vi "Add Correction.vi"(8 "error in (no error)":errorcluster, 9 "Type of Hexaboard":T1, 10 "XYZTheta":dbl[](array[numeric]), 11 "Carrier Tray in":refnum<class "Assembly Tray.lvclass">) -> (0 "error out":errorcluster, 2 "XYZTheta Out":dbl[](array[numeric]), 3 "Carrier Tray out":refnum<class "Assembly Tray.lvclass">)   [LabVIEW 2021, in "Assembly Tray.lvclass"]
uses:
  Assembly Tray.lvclass
  C:/Users/hep/Documents/UCSB-CMU-GantryCode/UCSB-Gantry-HEP-main (3)/UCSB-Gantry-HEP-main/Classes/Workspace/Fixture.lvclass
  Routine/TypeOfHexaboard.ctl
  Fixture.lvclass/Fixture.ctl
  Read Fixture ID.vi
  Read Position.vi
  Routine/Routine.lvclass
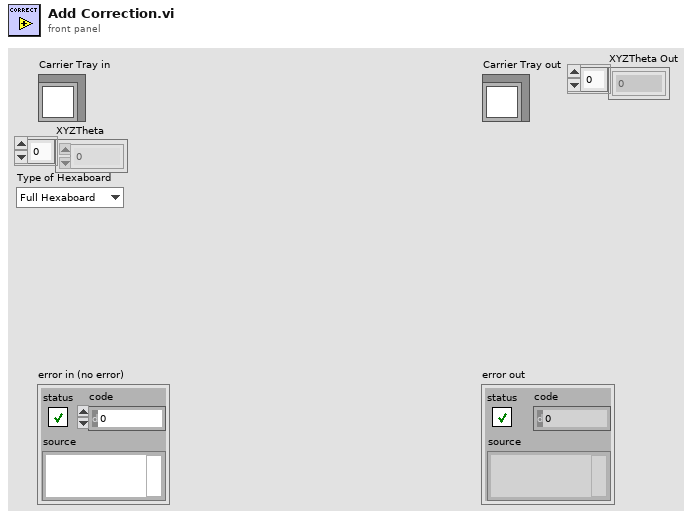
[diagram p1: front panel]
types:
  T1 = typedef "Routine.lvclass/TypeOfHexaboard.ctl" = enum16{"Full Hexaboard", "Right Partial PCB", "Right Partial Sensor", "Al Dummy Right Partial Sensor"}
  T2 = typedef "File Paths.ctl" = cluster{"Glue Pattern Folder":path, "Carrier Tray Folder":path, "Pick Up Tool Fixture Folder":path, "Components Folder":path, "Bellows Tool Offset.txt":path, "Pick Up Tool Offset.txt":path, "Dispense Tip Offset.txt":path, "Log Files":path, "Gantry Assembly Map.txt":path, "Syringe and offset map.txt":path}
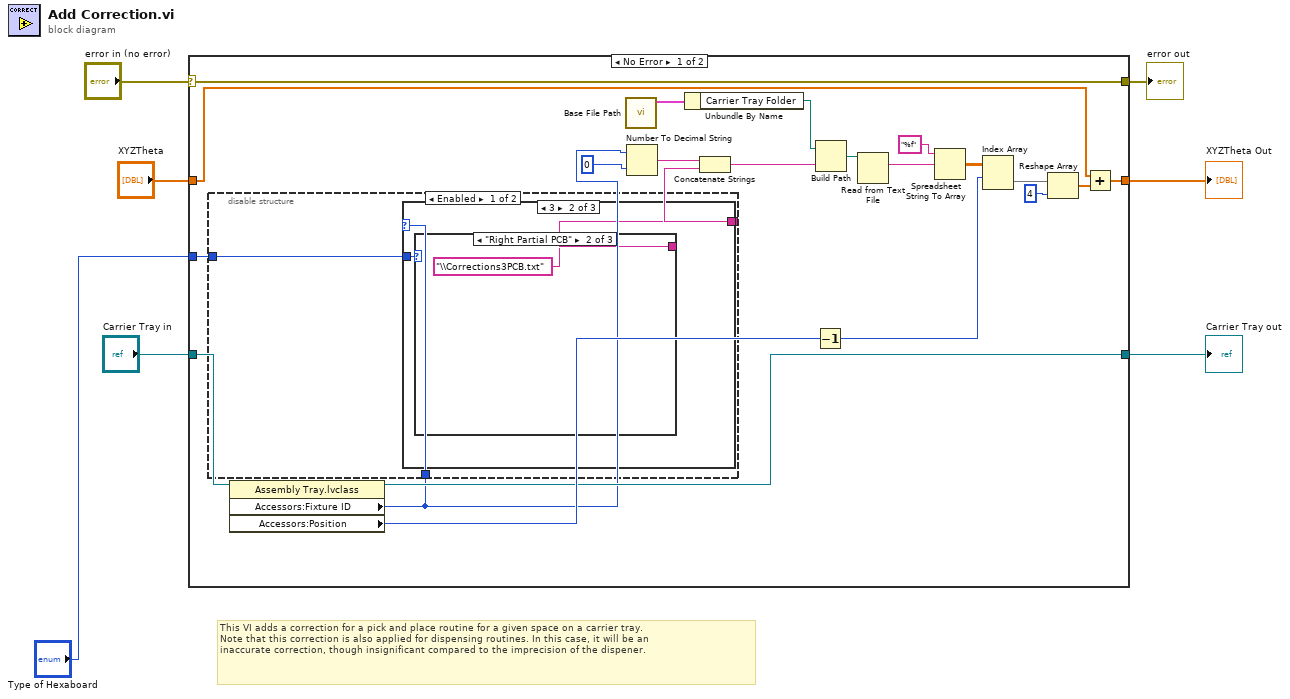
[diagram p0: block diagram]
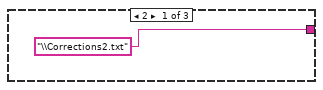
[diagram p2: hidden frame]
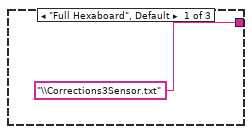
[diagram p3: hidden frame]
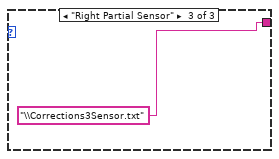
[diagram p4: hidden frame]
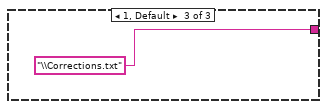
[diagram p5: hidden frame]
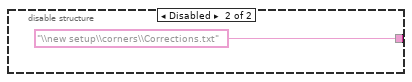
[diagram p6: hidden frame]
diagram:
  # "This VI adds a correction for a pick and place routine for a given space on a carrier tray.\nNote that this correction is also applied for dispensing routines. In this case, it will be an\ninaccurate correction, though insignificant compared to the imprecision of the dispener."
  n1 = case shown="No Error" "error in (no error)" {
    selector: "error in (no error)" -> [w29 w43]
    tunnel: [w29 w43] -> w6
    tunnel: [w10 w42] -> w4
    tunnel: "Carrier Tray in" -> [w12 w42]
    tunnel: "XYZTheta" -> [w15 w41]
    tunnel: [w13 w41] -> w2
    tunnel: "Type of Hexaboard" -> [w8 _]
    frame No Error {
      n2 = property class="Assembly Tray.lvclass"(reference=w12) -> (reference out=w10:refnum<class "Assembly Tray.lvclass">, "Accessors:Fixture ID"=w9:i32, "Accessors:Position"=w11:i32)  [unwired: 1 in, 1 out]
      n3 = disable-structure shown="Enabled" {
        disable-tunnel: [w32 "\\new setup\\corners\\Corrections.txt" ("name or relative path")] -> w24
        disable-tunnel: w9 -> [w31 _]
        disable-tunnel: w8 -> [w30 _]
        frame Enabled {
          n4 = case shown="3" w31 {
            tunnel: ["\\Corrections2.txt" ("name or relative path") w35 "\\Corrections.txt" ("name or relative path")] -> w32
            tunnel: w30 -> [_ w34 _]
            frame 2 {
            }
            frame 3 {
              n5 = case shown="\"Right Partial PCB\"" w34 {
                tunnel: ["\\Corrections3Sensor.txt" ("name or relative path") "\\Corrections3PCB.txt" ("name or relative path") "\\Corrections3Sensor.txt" ("name or relative path")] -> w35
                frame "Full Hexaboard", Default {
                }
                frame "Right Partial PCB" {
                }
                frame "Right Partial Sensor" {
                }
              }
            }
            frame 1, Default {
            }
          }
        }
        frame Disabled {
        }
      }
      n6 = call "Base File Path.vi"() -> ("Paths Out"=w28:T2)  [unwired: 11 in]
      n7 = Number To Decimal String(number=w9, width (-)=i16 0) -> (decimal integer string=w25:string)
      n8 = Unbundle By Name(w28) -> ("Carrier Tray Folder"=w27:path)
      n9 = Concatenate Strings(w25, w24) -> (w23:string)
      n10 = Decrement(x=w11) -> (x-1=w18:i32)
      n11 = Build Path(base path=w27, name or relative path=w23) -> (appended path=w22:path)
      n12 = Read from Text File(file (use dialog)=w22) -> (text=w21:string)  [unwired: 3 in, 3 out]
      n13 = Spreadsheet String To Array(format string="%f", spreadsheet string=w21) -> (array=w19:dbl[][])  [unwired: 2 in]
      n14 = Index Array(array=w19, index (row)=w18) -> (element=w16:dbl[])  [unwired: 1 in]
      n15 = Reshape Array(w16, 4 ("dimension size")) -> (w14:dbl[])
      n16 = Add(x=w15, y=w14) -> (x+y=w13:dbl[])
    }
    frame Error {
    }
  }
  "error out" <- w6
  "Carrier Tray out" <- w4
  "XYZTheta Out" <- w2
